vi "Problem 15 - backtracking-first working implementation.vi"(8 "error in (no error)":errorcluster) -> (0 "error out":errorcluster)   [LabVIEW 2021, in "Project Euler.lvlib"]
uses:
  Project Euler.lvlib
  lattice_path_node.ctl
  lattice_path_direction.ctl
  Utilities/Named Timers/Named Timers.lvlib
  Utilities/Named Counters/Named Counters.lvlib
panel:
  out "to_find_a_route (ms)":u32
  out "all paths":T1[][](array[typedef])
  out "current_path":T1[](array[typedef])
  out "no_of_routes":i32
  in  "destination":T1={"position"={"i"=2, "j"=2}, "unexplored children"=[]}
  in  "start":T1={"position"={"i"=0, "j"=0}, "unexplored children"=[enum."to the right", enum."downwards"]}
  out "Loop iteration":i32
  in  "Dev: stop early":bool
  out "no. of columns":i32
  out "no. of rows":i32
  out "map\n2D array of nodes\n(n+1) x (n+1) size":T1[][](array[typedef])
  out "j":i32
  out "i":i32
  in  "n":i32=20
  out "Answer":string
  out "Total execution time (ms)":u32
  # "Input\nInputs to the VI"
  # "Development\nControls or indicators that are useful for development or testing, but which are not outputs of the VI."
  # "Output\nOutputs of the VI"
  # "First implementation:\n\n20x20 grid (21 nodex x 21 nodes):\n125,059 routes found in 506,856 ms -> 4.05 ms to find one route (one average)"
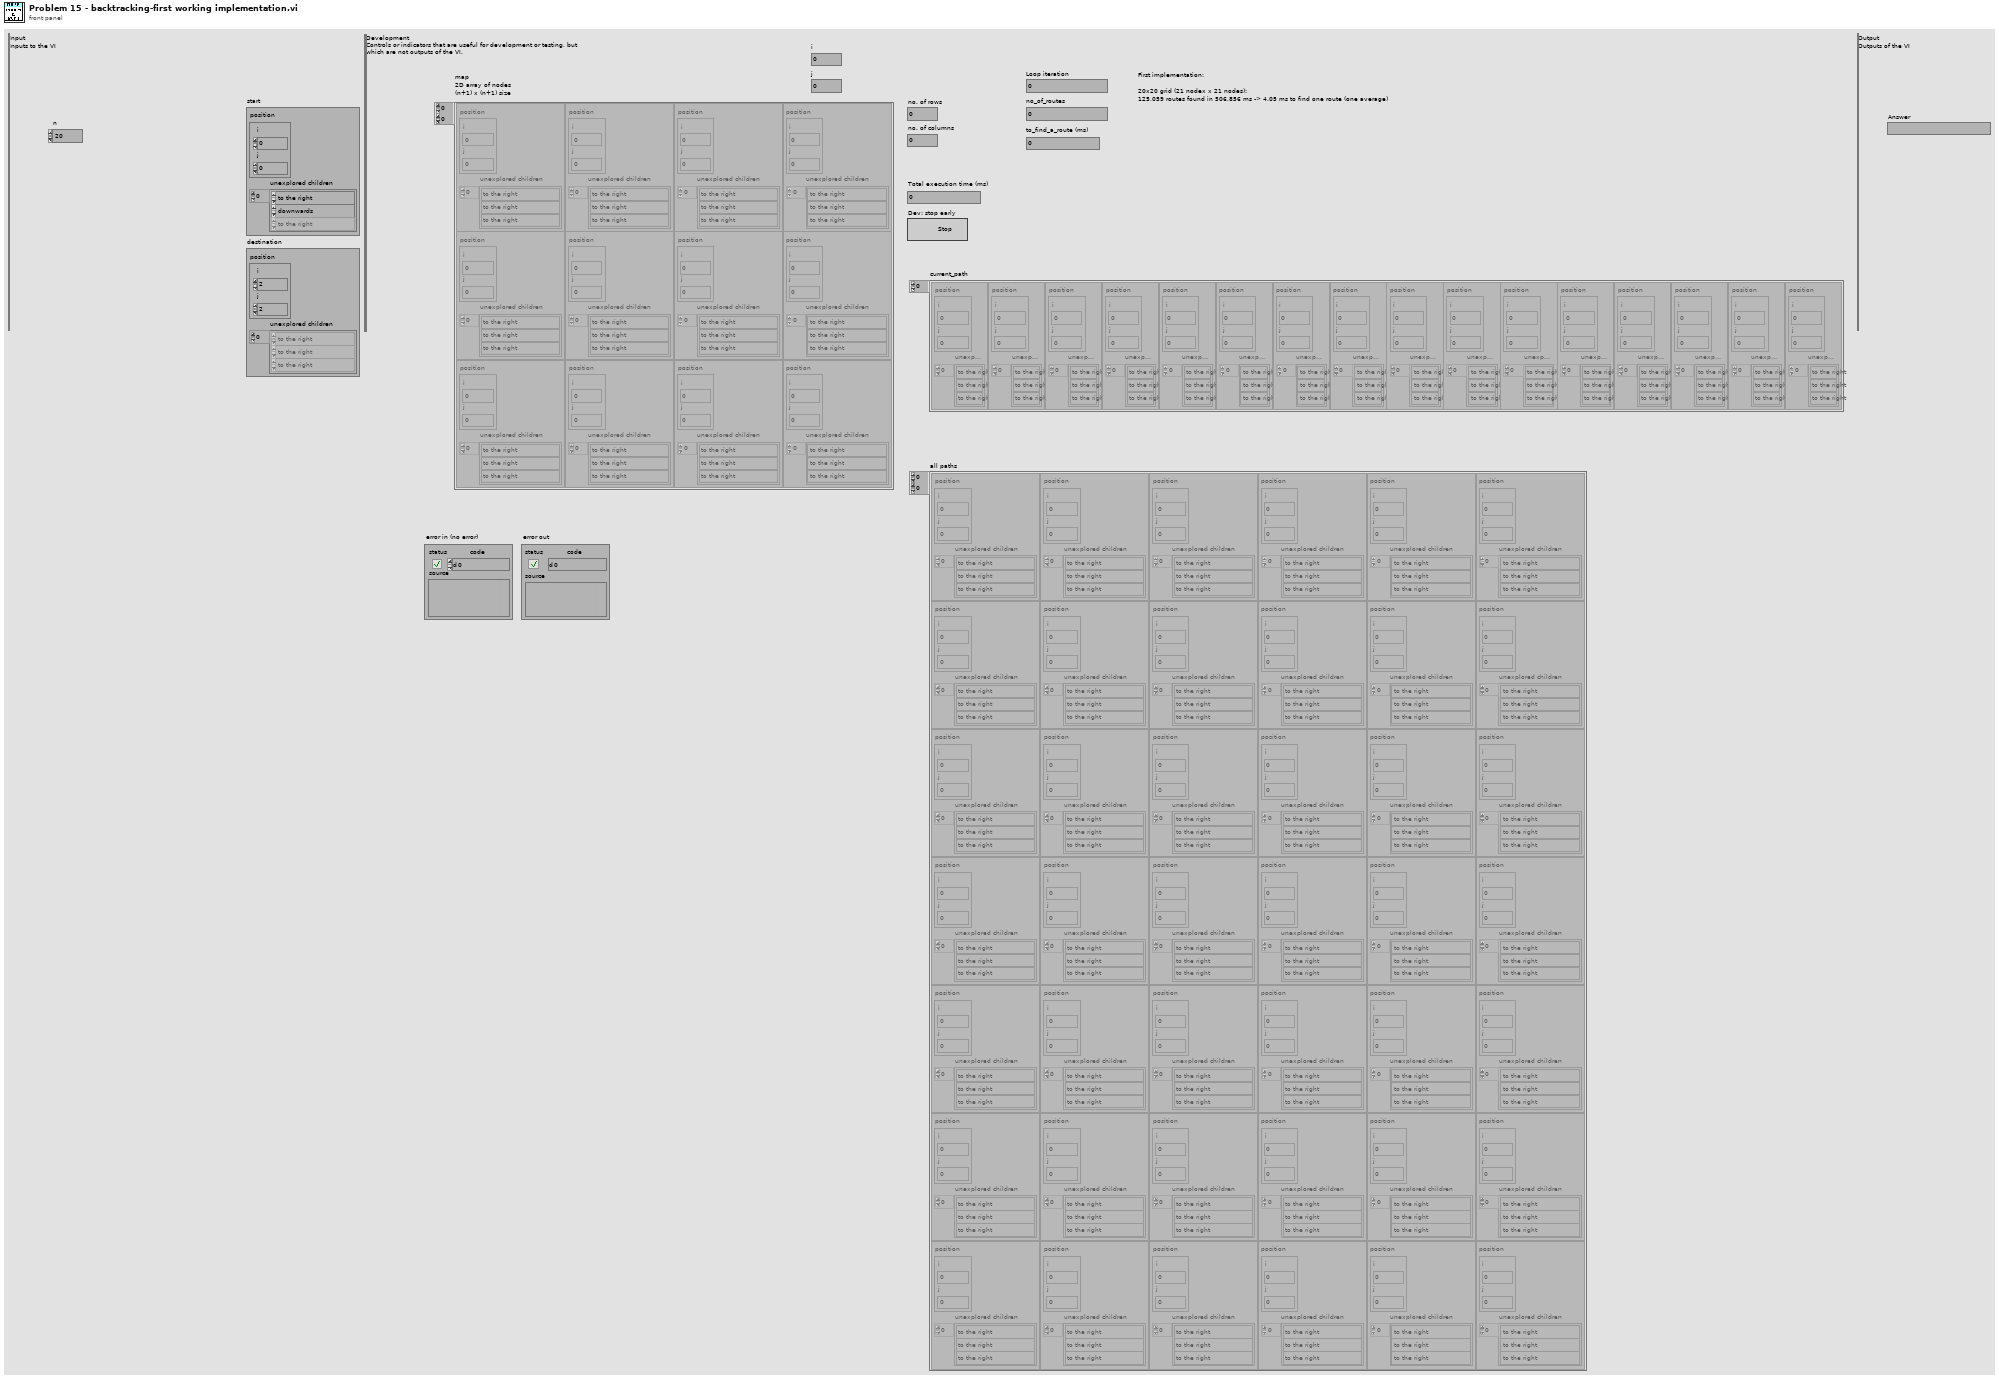
[diagram p1: front panel]
types:
  T1 = typedef "Project Euler.lvlib/lattice_path_node.ctl" = cluster{"position":cluster{"i":i32, "j":i32}, "unexplored children":T2[]}
  T2 = typedef "Project Euler.lvlib/lattice_path_direction.ctl" = enum16{"to the right", "downwards"}
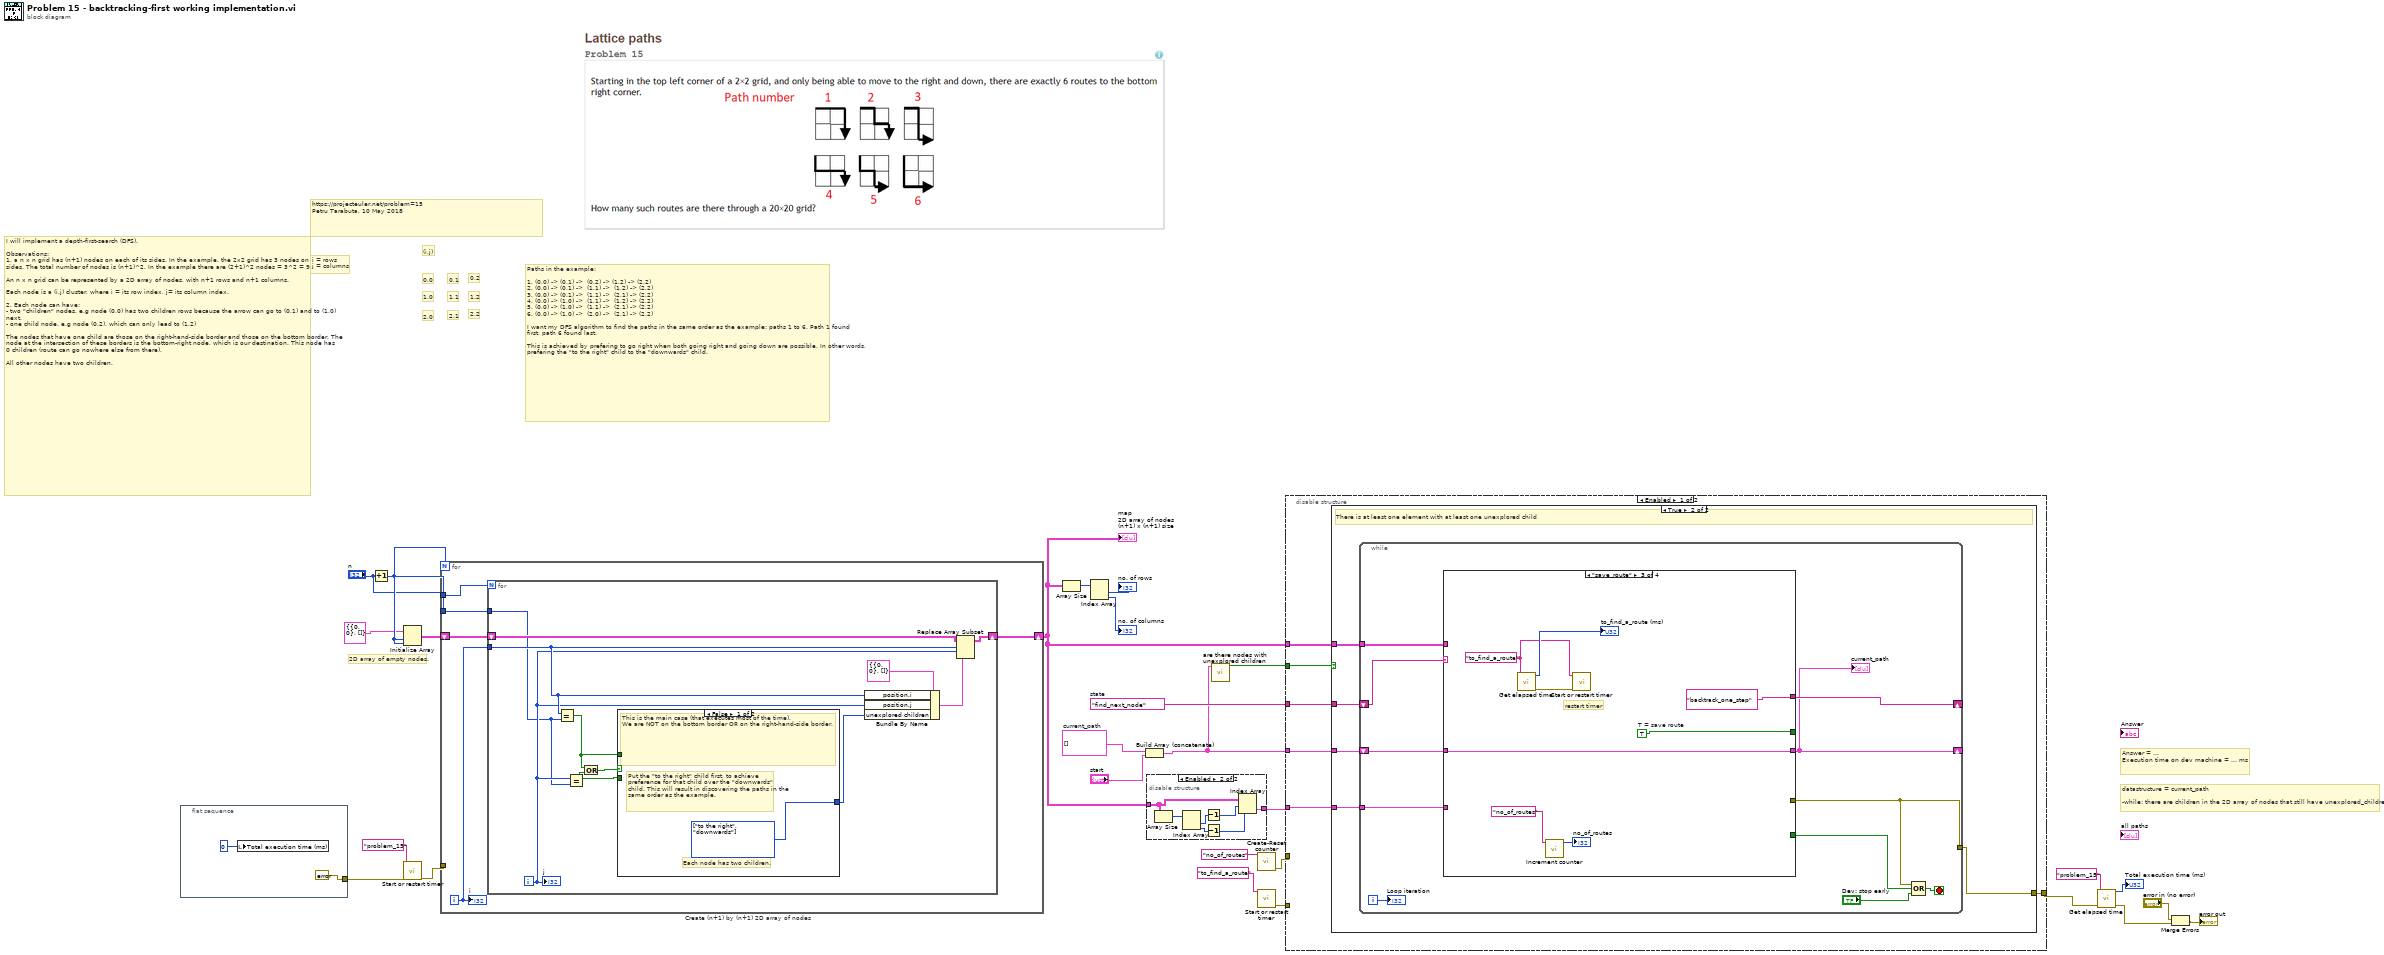
[diagram p0: block diagram]
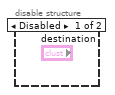
[diagram p2: hidden frame]
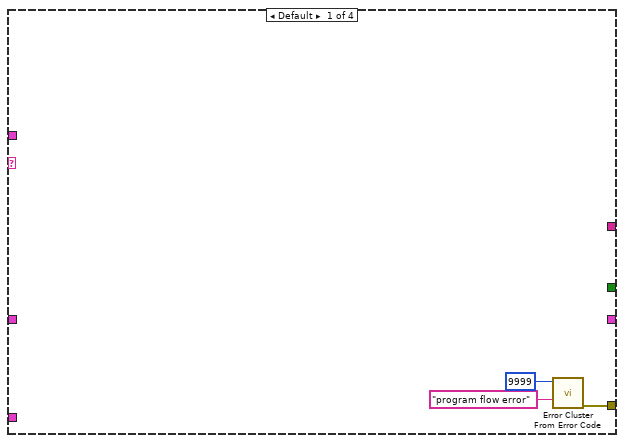
[diagram p4: hidden frame]
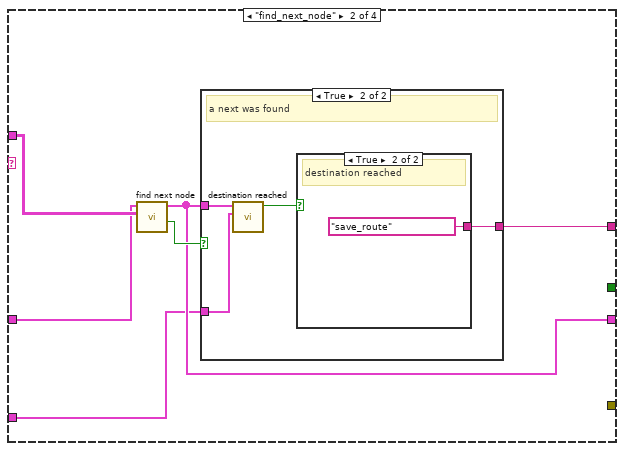
[diagram p5: hidden frame]
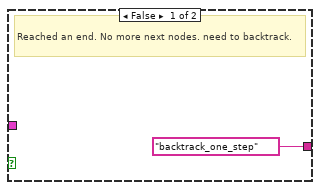
[diagram p6: hidden frame]
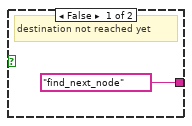
[diagram p7: hidden frame]
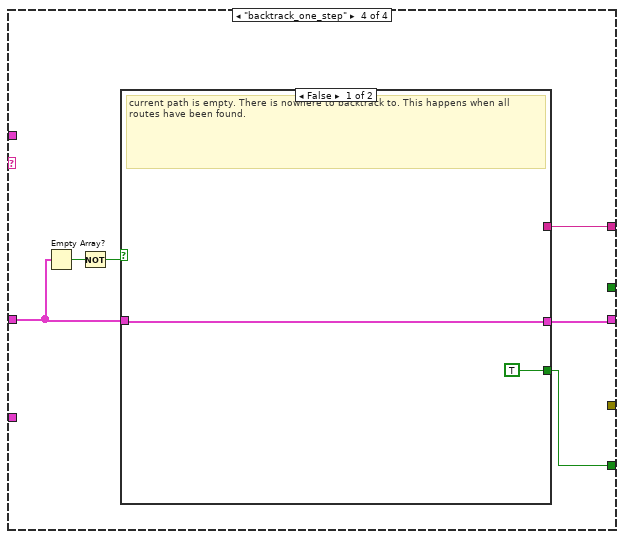
[diagram p8: hidden frame]
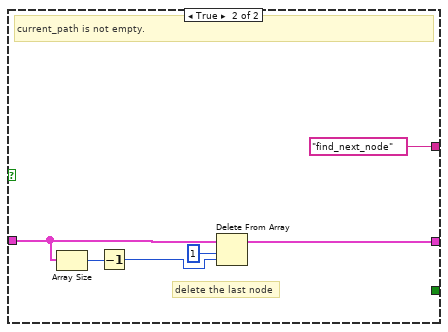
[diagram p9: hidden frame]
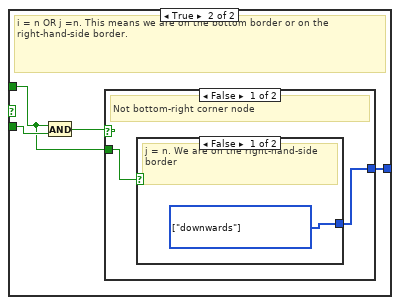
[diagram p11: hidden frame]
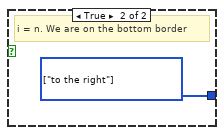
[diagram p12: hidden frame]
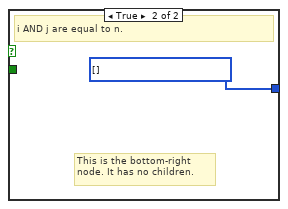
[diagram p13: hidden frame]
diagram:
  w12 = "find_next_node"  # state
  w13 = T1[] []  # current_path
  # "datastructure = current_path\n\n-while: there are children in the 2D array of nodes that still have unexplored_children"
  # "2D array of empty nodes."
  # "Paths in the example:\n\n1. (0,0) -> (0,1) ->  (0,2) -> (1,2) -> (2,2)\n2. (0,0) -> (0,1) ->  (1,1) ->  (1,2) -> (2,2)\n3. (0,0) -> (0,1) ->  (1,1) ->  (2,1) -> (2,2)\n4. (0,0) -> (1,0) ->  (1,1) ->  (1,2) -> (2,2)\n5. (0,0) -> (1,0) ->  (1,1) ->  (2,1) -> (2,2)\n6. (0,0) -> (1,0) ->  (2,0) ->  (2,1) -> (2,2)\n\nI want my DFS algorithm to find the paths in the same order as the example: paths 1 to 6. Path 1 found first, path 6 found last.\n\nThis is achieved by prefering to go right when both going right and going down are possible. In other words, prefering the \"to the right\" child to the \"downwards\" child."
  # "2,2"
  # "2,1"
  # "1,2"
  # "1,1"
  # "0,2"
  # "0,1"
  # "2,0"
  # "(i,j)"
  # "i = rows\nj = columns"
  # "1,0"
  # "0,0"
  # "I will implement a depth-first-search (DFS).\n\nObservations:\n1. a n x n grid has (n+1) nodes on each of its sides. In the example, the 2x2 grid has 3 nodes on each of its sides. The total number of nodes is (n+1)^2. In the example there are (2+1)^2 nodes = 3^2 = 9 nodes\n\nAn n x n grid can be represented by a 2D array of nodes, with n+1 rows and n+1 columns.\n\nEach node is a (i,j) cluster, where i = its row index, j= its column index.\n\n2. Each node can have:\n- two \"children\" nodes. e.g node (0,0) has two children rows because the arrow can go to (0,1) and to (1,0) next.\n- one child node. e.g node (0,2), which can only lead to (1,2)\n\nThe nodes that have one child are those on the right-hand-side border and those on the bottom border. The node at the intersection of these borders is the bottom-right node, which is our destination. This node has 0 children (route can go nowhere else from there).\n\nAll other nodes have two children."
  # "Answer = ... \nExecution time on dev machine = ... ms"
  # "https://projecteuler.net/problem=15\nPetru Tarabuta, 10 May 2018"
  n1 = flat-sequence {
    tunnel: [w28] -> _
    tunnel: [w28] -> w14
    frame #0 {
      w28 = errorcluster {"status"=FALSE, "code"=0, "source"=""} ("error constant")
      n2 = local write "Total execution time (ms)"(u32 0 ("Total execution time (ms)")) -> ()
    }
  }
  n3 = Increment(x="n") -> (x+1=w25:i32)
  n4 = Initialize Array(T1 {"position"={"i"=0, "j"=0}, "unexplored children"=[]} ("node"), w25, w25) -> (w23:T1[][])
  n5 = call "Start or restart timer.vi"("error in (no error)"=w14, "Timer name"="problem_15") -> ("error out"=w17:errorcluster)  [unwired: 9 in]
  n6 = for "Create (n+1) by (n+1) 2D array of nodes" {
    N: w25 -> [_]
    tunnel: w25 -> [w34]
    shift-right: [w31] -> w4
    shift-left: w23 -> [w33]
    tunnel: "n" -> [w30]
    tunnel: w17 -> [_]
    i -> [w32]
    n7 = for {
      N: w34 -> [_]
      tunnel: w32 -> [w41]
      shift-right: [w42] -> w31
      shift-left: w33 -> [w45]
      tunnel: w30 -> [w39]
      i -> [w40]
      n8 = Equal?(x=w41, y=w39) -> (x = y?=w36:bool)
      n9 = Equal?(x=w40, y=w39) -> (x = y?=w35:bool)
      n10 = Compound Arithmetic op=OR(w36, w35) -> (w38:bool)
      n11 = case shown="False" w38 {
        tunnel: [w46 w48] -> w37
        tunnel: w36 -> [_ w47]
        tunnel: w35 -> [_ w50]
        frame False {
          w46 = T2[] [enum."to the right", enum."downwards"] items=["to the right", "downwards"] ("children")
          # "Put the \"to the right\" child first, to achieve preference for that child over the \"downwards\" child. This will result in discovering the paths in the same order as the example."
          # "Each node has two children."
          # "This is the main case (that executes most of the time).\nWe are NOT on the bottom border OR on the right-hand-side border."
        }
        frame True {
          # "i = n OR j =n. This means we are on the bottom border or on the right-hand-side border."
          n12 = And(x=w47, y=w50) -> (x .and. y?=w49:bool)
          n13 = case shown="False" w49 {
            tunnel: [w51 w55] -> w48
            tunnel: w47 -> [w52 _]
            frame False {
              # "Not bottom-right corner node"
              n14 = case shown="False" w52 {
                tunnel: [w53 w54] -> w51
                frame False {
                  w53 = T2[] [enum."downwards"] items=["to the right", "downwards"] ("children")
                  # "j = n. We are on the right-hand-side border"
                }
                frame True {
                  w54 = T2[] [enum."to the right"] items=["to the right", "downwards"] ("children")
                  # "i = n. We are on the bottom border"
                }
              }
            }
            frame True {
              w55 = T2[] [] items=["to the right", "downwards"] ("children")
              # "This is the bottom-right node. It has no children."
              # "i AND j are equal to n."
            }
          }
        }
      }
      n15 = Bundle By Name(cluster=T1 {"position"={"i"=0, "j"=0}, "unexplored children"=[]} ("node"), "position.i"=w41, "position.j"=w40, "unexplored children"=w37) -> (w43:T1)
      n16 = Replace Array Subset(array=w45, new element=w43, index (row)=w41, index (col)=w40) -> (w42:T1[][])
      "j" <- w40
    }
    "i" <- w32
  }
  "map\n2D array of nodes\n(n+1) x (n+1) size" <- w4
  n17 = Array Size(array=w4) -> (size(s)=w21:i32[])
  n18 = Index Array(array=w21) -> (element #1=→"no. of rows":i32, element #2=→"no. of columns":i32)  [unwired: 2 in]
  n19 = Build Array (concatenate)(w13, "start") -> (w7:T1[])
  n20 = disable-structure shown="Enabled" {
    disable-tunnel: w4 -> [_ w61]
    disable-tunnel: [_ w56] -> w3
    frame Disabled {
    }
    frame Enabled {
      n21 = Array Size(array=w61) -> (size(s)=w62:i32[])
      n22 = Index Array(array=w62) -> (element #1=w60:i32, element #2=w58:i32)  [unwired: 2 in]
      n23 = Decrement(x=w60) -> (x-1=w59:i32)
      n24 = Decrement(x=w58) -> (x-1=w57:i32)
      n25 = Index Array(array=w61, index (row)=w59, index (col)=w57) -> (element=w56:T1)
    }
  }
  n26 = call "are there nodes with unexplored children.vi"("current_path"=w7) -> ("T = there is at least one node with at least one unexplored child"=w18:bool)  [unwired: 9 in, 1 out]
  n27 = call "Create-Reset counter.vi"("Counter name (dflt=blank)"="no_of_routes") -> ("error out"=w5:errorcluster)  [unwired: 10 in]
  n28 = call "Start or restart timer.vi"("Timer name"="to_find_a_route") -> ("error out"=w1:errorcluster)  [unwired: 10 in]
  n29 = disable-structure shown="Enabled" {
    disable-tunnel: w18 -> [w68 _]
    disable-tunnel: w4 -> [w67 _]
    disable-tunnel: [w66 _] -> w15
    disable-tunnel: w12 -> [w65 _]
    disable-tunnel: w7 -> [w64 _]
    disable-tunnel: w3 -> [w63 _]
    disable-tunnel: w5 -> [_ _]
    disable-tunnel: w1 -> [_ _]
    frame Enabled {
      n30 = case shown="True" w68 {
        tunnel: w67 -> [_ w73]
        tunnel: [_ w70] -> w66
        tunnel: w64 -> [_ w72]
        tunnel: w65 -> [_ w71]
        tunnel: w63 -> [_ w69]
        frame False {
        }
        frame True {
          # "There is at least one element with at least one unexplored child"
          n31 = while {
            shift-right: [w75] -> _
            shift-left: w72 -> [w79]
            shift-right: [w78] -> _
            shift-left: w71 -> [w77]
            tunnel: [w81] -> w70
            tunnel: w73 -> [w80]
            tunnel: w69 -> [w76]
            i -> [w82]
            stop <- w83 stop-if-true
            n32 = case shown="\"save_route\"" w77 {
              tunnel: [w85 _ _ _] -> w81
              tunnel: w80 -> [_ w93 _ _]
              tunnel: w79 -> [_ w92 w108 w112]
              tunnel: [_ w90 "backtrack_one_step" w110] -> w78
              tunnel: [_ w89 w108 w111] -> w75
              tunnel: w76 -> [_ w88 _ _]
              tunnel: [_ _ w107 _] -> _
              tunnel: [_ _ _ w109] -> w74
              frame Default {
                n33 = call <vilib>:"Error Cluster From Error Code.vi"("error message (\"\")"="program flow error" ("error message (\"\")"), "error code (0)"=9999) -> ("error out"=w85:errorcluster)  [unwired: 7 in]
              }
              frame "find_next_node" {
                n34 = call "find next node.vi"("map"=w93, "current_path in"=w92) -> ("T = a next node was found"=w91:bool, "current_path out"=w89:T1[])  [unwired: 6 in, 2 out]
                n35 = case shown="True" w91 {
                  tunnel: w89 -> [_ w98]
                  tunnel: ["backtrack_one_step" w96] -> w90
                  tunnel: w88 -> [_ w95]
                  frame False {
                    # "Reached an end. No more next nodes. need to backtrack."
                  }
                  frame True {
                    # "a next was found"
                    n36 = call "destination reached.vi"("destination"=w95, "current_path"=w98) -> ("T = destination has been reached"=w97:bool)  [unwired: 8 in, 1 out]
                    n37 = case shown="True" w97 {
                      tunnel: ["find_next_node" "save_route"] -> w96
                      frame False {
                        # "destination not reached yet"
                      }
                      frame True {
                        # "destination reached"
                      }
                    }
                  }
                }
              }
              frame "save_route" {
                w101 = "to_find_a_route" ("Timer name")
                w107 = TRUE  # T = save route
                # "restart timer"
                n38 = call "Get elapsed time.vi"("Timer name"=w101) -> ("error out"=w102:errorcluster, "Elapsed time (ms)"=→"to_find_a_route (ms)":u32)  [unwired: 7 in, 2 out]
                n39 = call "Increment counter.vi"("Counter name (dflt=blank)"="no_of_routes") -> ("Value (after increment)"=→"no_of_routes":i32)  [unwired: 9 in, 1 out]
                n40 = call "Start or restart timer.vi"("error in (no error)"=w102, "Timer name"=w101) -> ()  [unwired: 9 in, 1 out]
              }
              frame "backtrack_one_step" {
                n41 = Empty Array?(array=w112) -> (empty?=w114:bool)
                n42 = Not(x=w114) -> (.not. x?=w113:bool)
                n43 = case shown="False" w113 {
                  tunnel: w112 -> [w116 w121]
                  tunnel: [w116 w118] -> w111
                  tunnel: [_ "find_next_node"] -> w110
                  tunnel: [TRUE _] -> w109
                  frame False {
                    # "current path is empty. There is nowhere to backtrack to. This happens when all routes have been found."
                  }
                  frame True {
                    # "delete the last node"
                    # "current_path is not empty."
                    n44 = Array Size(array=w121) -> (size(s)=w120:i32)
                    n45 = Decrement(x=w120) -> (x-1=w119:i32)
                    n46 = Delete From Array(array=w121, length=1, index=w119) -> (array with subset deleted=w118:T1[])  [unwired: 1 out]
                  }
                }
              }
            }
            "current_path" <- w75
            n47 = Compound Arithmetic op=OR(w81, w74, "Dev: stop early") -> (w83:bool)
            "Loop iteration" <- w82
          }
        }
      }
    }
    frame Disabled {
    }
  }
  n48 = call "Get elapsed time.vi"("error in (no error)"=w15, "Timer name"="problem_15") -> ("error out"=w9:errorcluster, "Elapsed time (ms)"=→"Total execution time (ms)":u32)  [unwired: 6 in, 2 out]
  n49 = Merge Errors("error in (no error)", w9) -> (→"error out":errorcluster)
